vi "application_path.vi"() -> (1 "path":path)   [LabVIEW 2018]
doc: "Vi for determing current application path.\ncode snippet from:\nhttps://knowledge.ni.com/KnowledgeArticleDetails?id=kA00Z0000019NFfSAM"
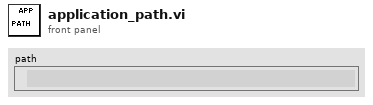
[diagram p1: front panel]
types:
  T1 = enum32{"invalid app kind", "Development System", "Run Time System", "Student Edition", "Embedded LabVIEW", "Evaluation", "Custom"}
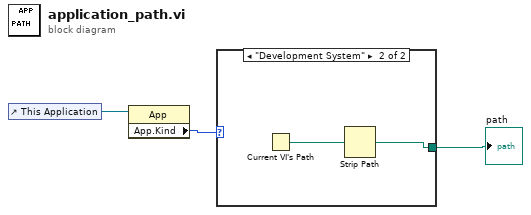
[diagram p0: block diagram]
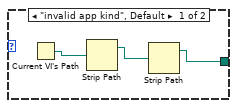
[diagram p2: hidden frame]
diagram:
  n1 = control-ref of="This Application"() -> (w1:refnum<vi>)
  n2 = property class="App"(reference=w1) -> ("App.Kind"=w3:T1)  [unwired: 1 in, 2 out]
  n3 = case shown="\"Development System\"" w3 {
    tunnel: [w4 w7] -> w2
    frame "invalid app kind", Default {
      n4 = Current VI's Path() -> (path=w6:path)
      n5 = Strip Path(path=w6) -> (stripped path=w5:path)  [unwired: 1 out]
      n6 = Strip Path(path=w5) -> (stripped path=w4:path)  [unwired: 1 out]
    }
    frame "Development System" {
      n7 = Current VI's Path() -> (path=w8:path)
      n8 = Strip Path(path=w8) -> (stripped path=w7:path)  [unwired: 1 out]
    }
  }
  "path" <- w2
